vi "finishUp.vi"(8 "error in (no error)":errorcluster, 11 "ChangeValueAction in":refnum<class "ChangeValueAction.lvclass">) -> (0 "error out":errorcluster, 3 "ChangeValueAction out":refnum<class "ChangeValueAction.lvclass">)   [LabVIEW 2009, in "Views.lvlib" / "ScriptEditor.lvlib" / "ChangeValueAction.lvclass"]
uses:
  ChangeValueAction.lvclass
  ChangeValueAction.lvclass/ChangeValueAction.ctl
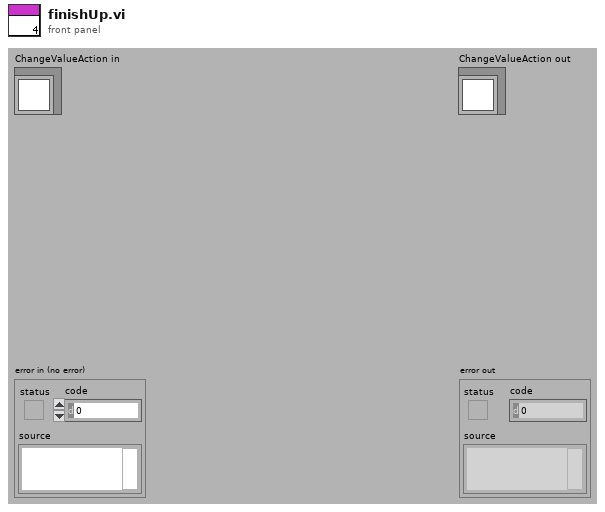
[diagram p1: front panel]
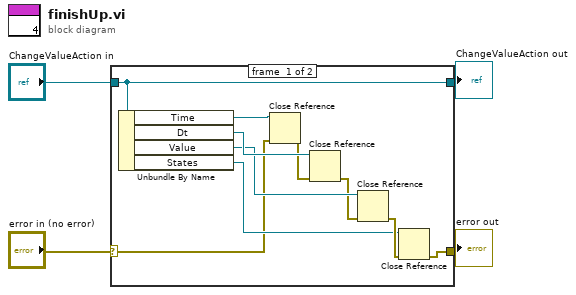
[diagram p0: block diagram]
diagram:
  n1 = case shown="No Error" "error in (no error)" {
    selector: "error in (no error)" -> [w5 w15]
    tunnel: "ChangeValueAction in" -> [w14 w16]
    tunnel: [w14 w16] -> w2
    tunnel: [w6 w15] -> w1
    frame #0 {
      n2 = Unbundle By Name(w14) -> ("Time"=w13:refnum<vi>, "Dt"=w12:refnum<vi>, "Value"=w11:refnum<vi>, "States"=w7:refnum<vi>)
      n3 = Close Reference(reference=w13, error in (no error)=w5) -> (error out=w10:errorcluster)
      n4 = Close Reference(reference=w12, error in (no error)=w10) -> (error out=w9:errorcluster)
      n5 = Close Reference(reference=w11, error in (no error)=w9) -> (error out=w8:errorcluster)
      n6 = Close Reference(reference=w7, error in (no error)=w8) -> (error out=w6:errorcluster)
    }
    frame #1 {
    }
  }
  "error out" <- w1
  "ChangeValueAction out" <- w2
